vi "Create.vi"(5 "Fact In":refnum<class "Fact.lvclass">, 8 "error in (no error)":errorcluster, 10 "VI Refnum":refnum<vi>) -> (0 "error out":errorcluster, 3 "Fact":refnum<class "Fact.lvclass">)   [LabVIEW 2019, in "Fact.lvclass"]
uses:
  Fact.lvclass
  Fact.lvclass/Fact.ctl
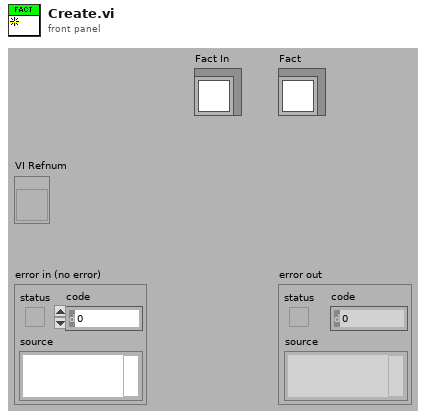
[diagram p1: front panel]
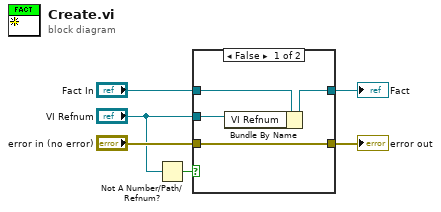
[diagram p0: block diagram]
diagram:
  n1 = Not A Number/Path/Refnum?(number/path/refnum="VI Refnum") -> (NaN/Path/Refnum?=w1:bool)
  n2 = case shown="False" w1 {
    tunnel: "error in (no error)" -> [w10 w11]
    tunnel: "Fact In" -> [w9 w12]
    tunnel: [w8 w12] -> w4
    tunnel: [w10 w11] -> w3
    tunnel: "VI Refnum" -> [w7 _]
    frame False {
      n3 = Bundle By Name(cluster=w9, "VI Refnum"=w7) -> (w8:refnum<class "Fact.lvclass">)
    }
    frame True {
    }
  }
  "error out" <- w3
  "Fact" <- w4
